vi "GOLPI full test.vi"() -> ()   [LabVIEW 2013, in "GOLPI library.lvlib"]
doc: "Makes test of all routines in GOLPI library. Good for testing changes in GOLPI library or testing compatibility with new versions of GNU Octave."
uses:
  GOLPI library.lvlib
  Set Variable - polymorph parts/Set Double.vi
  Get Variable - polymorph parts/Get Double.vi
  Set Variable - polymorph parts/Set Double Complex.vi
  Get Variable - polymorph parts/Get Double Complex.vi
  Set Variable - polymorph parts/Set 2D Array Double.vi
  Get Variable - polymorph parts/Get 2D Array Double.vi
  Set Variable - polymorph parts/Set 2D Array Double Complex.vi
  Get Variable - polymorph parts/Get 2D Array Double Complex.vi
  Set Variable - polymorph parts/Set String.vi
  Get Variable - polymorph parts/Get String.vi
  Set Variable - polymorph parts/Set 1D Array String.vi
  Get Variable - polymorph parts/Get 1D Array String.vi
panel:
  out "now running test no:":i32
  out "all tests result":bool
  out "test results":T1(array[cluster])
  in  "do tests with large random datasets?":bool
  out "GNU Octave version":string
  out "exit code":i32
  out "error out":errorcluster
  in  "Octave binary directory":path=path "C:/Program Files/Octave-3.6.2/bin"
  in  "Working directory":path=path "C:/"
  # "Runs various tests and checks all parts of GOLPI library.\nSelecting 'do tests with large random datasets' cause\nrunning of time consuming tests.\nIf all tests are OK, GOLPI is fully working with selected\nGNU Octave binary."
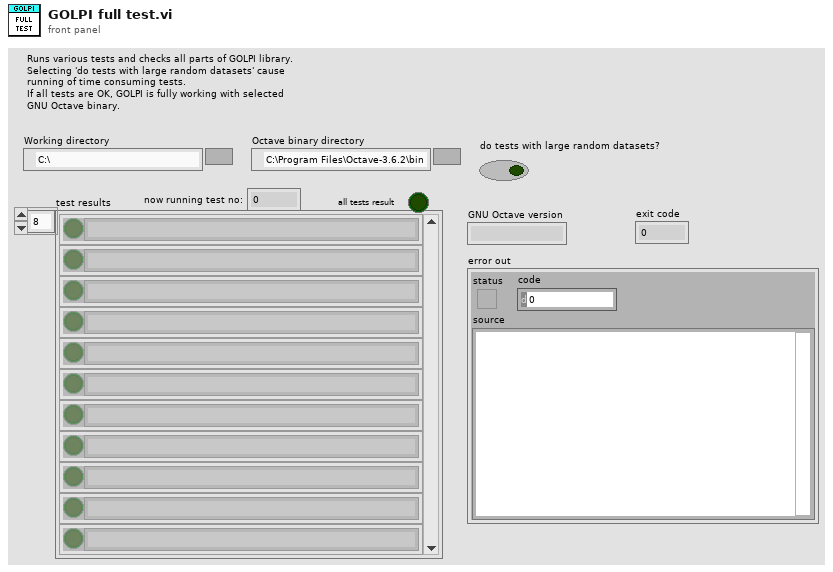
[diagram p1: front panel]
types:
  T1 = cluster{"test result":bool, "variable name":string}[]
  T2 = typedef "GOLPI library.lvlib/GOLPI reference Type Def.ctl" = cluster{"pipe handle":T3, "fast read timeout [ms]":u32, "fast read settle time [ms]":u32, "fast read to multiple [ms]":u32, "max elements per input line":u32, "slow read timeout [ms]":u32, "stdin double format specifier":string, "max elements per stdout output column":u32}
  T3 = typedef "LV Process library.lvlib/Pipe Handle.ctl" = cluster{"lv_proc.dll file path":path, "process instance handle":u32[]}
  T4 = cluster{"test result":bool, "variable name":string}
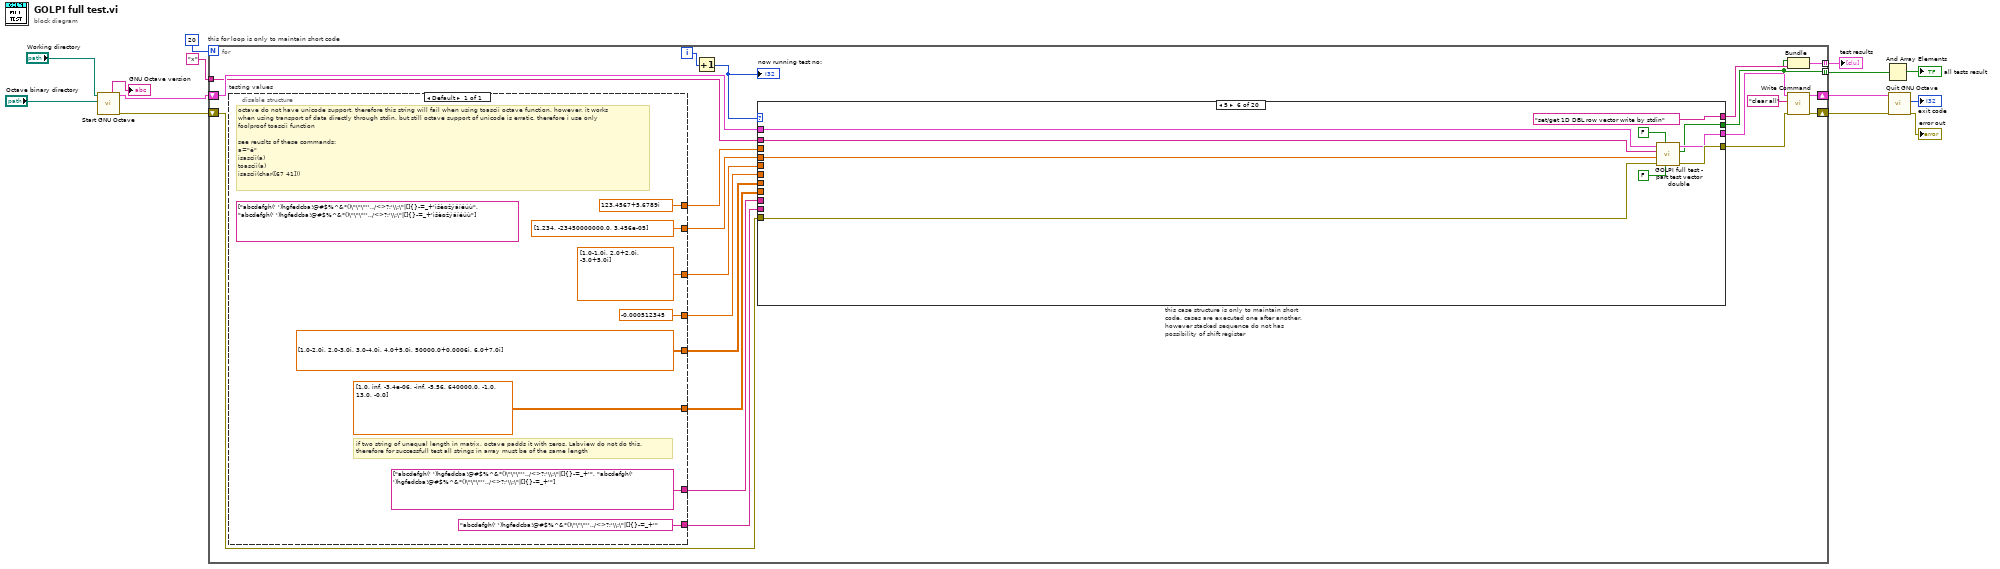
[diagram p0: block diagram]
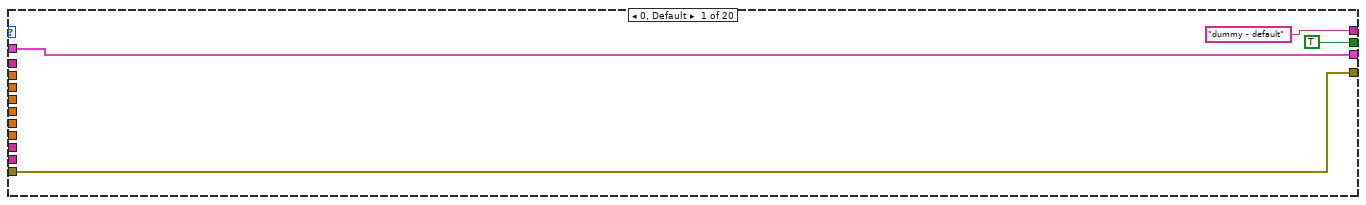
[diagram p2: hidden frame]
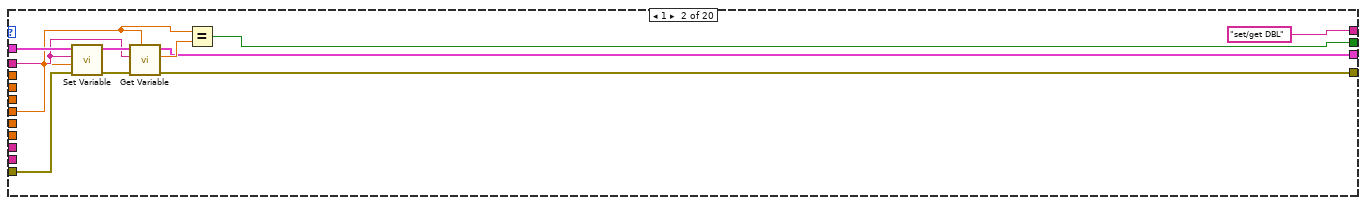
[diagram p3: hidden frame]
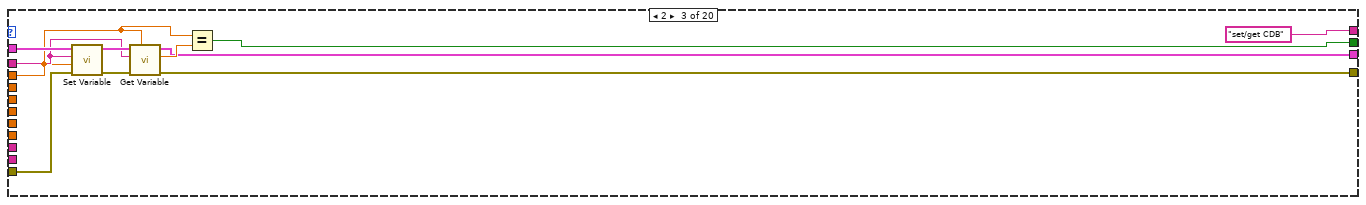
[diagram p4: hidden frame]
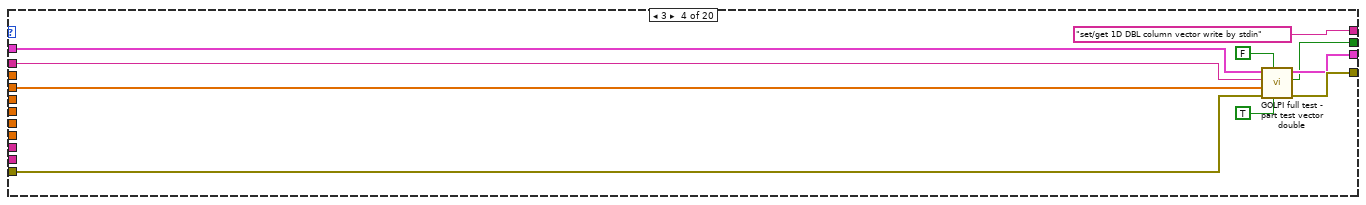
[diagram p5: hidden frame]
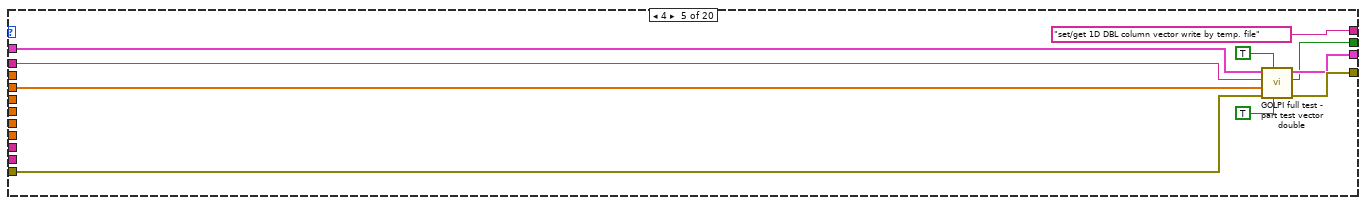
[diagram p6: hidden frame]
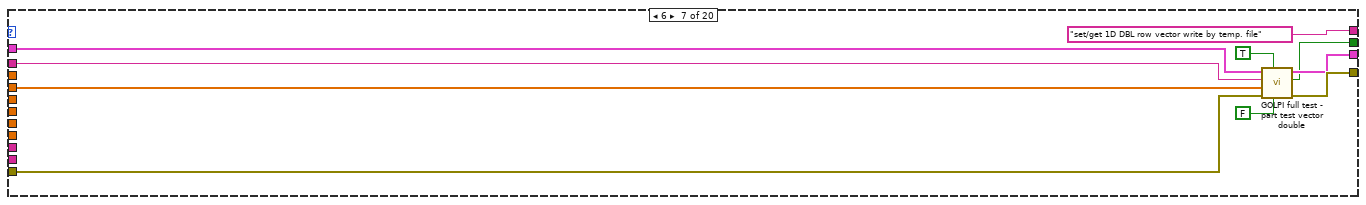
[diagram p7: hidden frame]
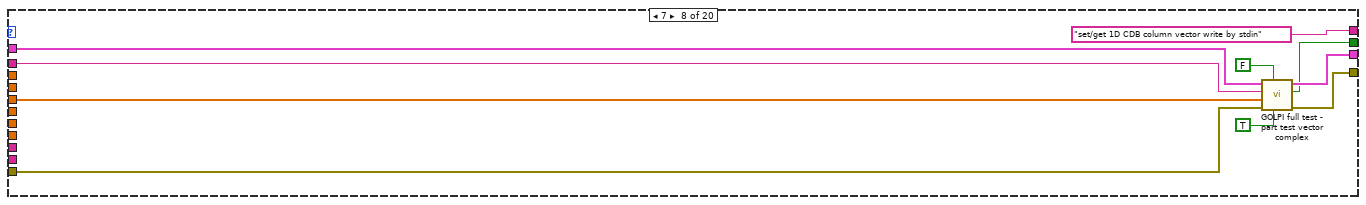
[diagram p8: hidden frame]
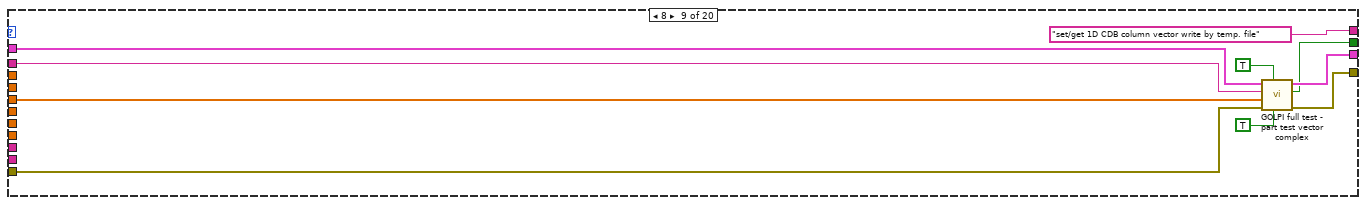
[diagram p9: hidden frame]
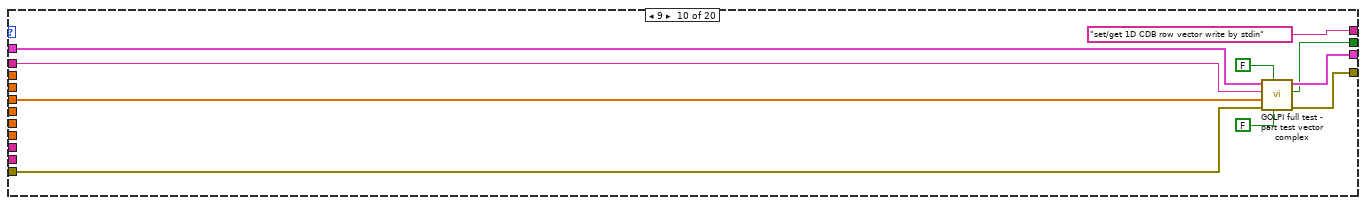
[diagram p10: hidden frame]
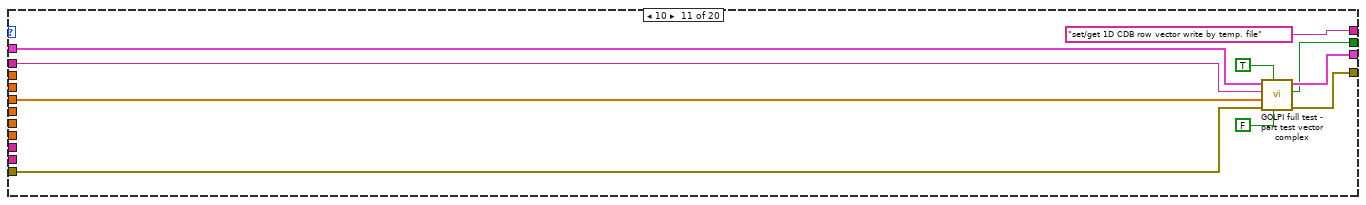
[diagram p11: hidden frame]
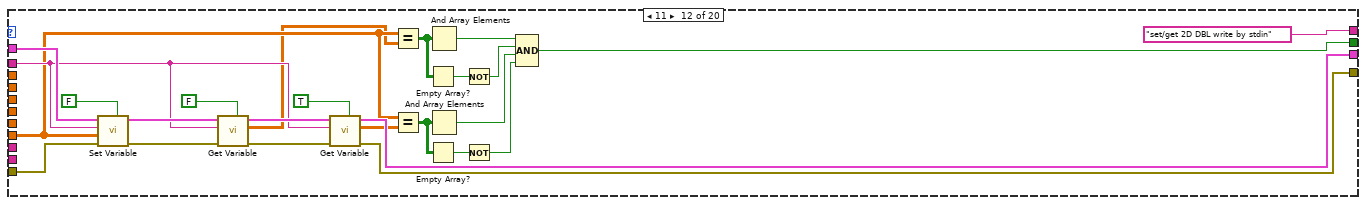
[diagram p12: hidden frame]
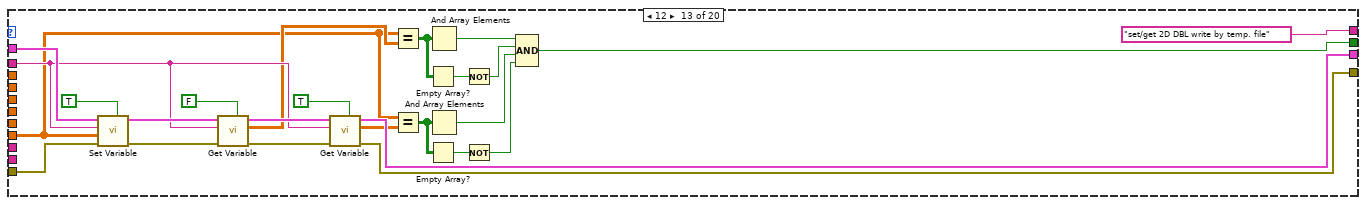
[diagram p13: hidden frame]
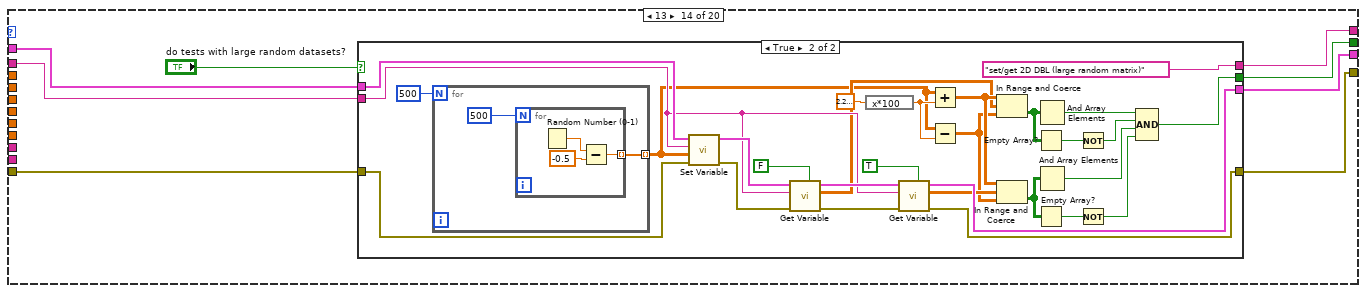
[diagram p14: hidden frame]
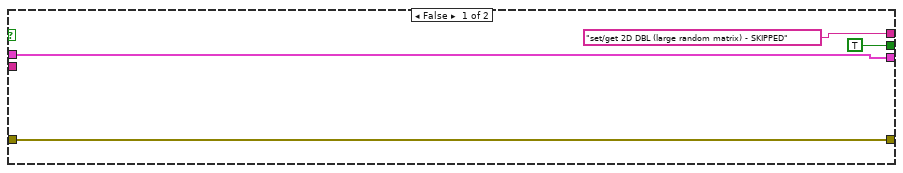
[diagram p15: hidden frame]
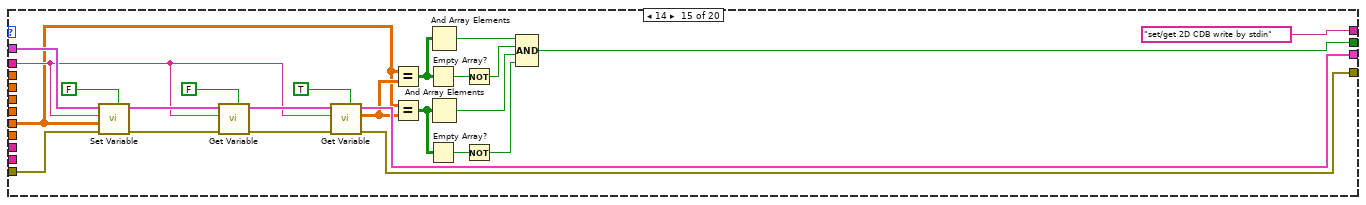
[diagram p16: hidden frame]
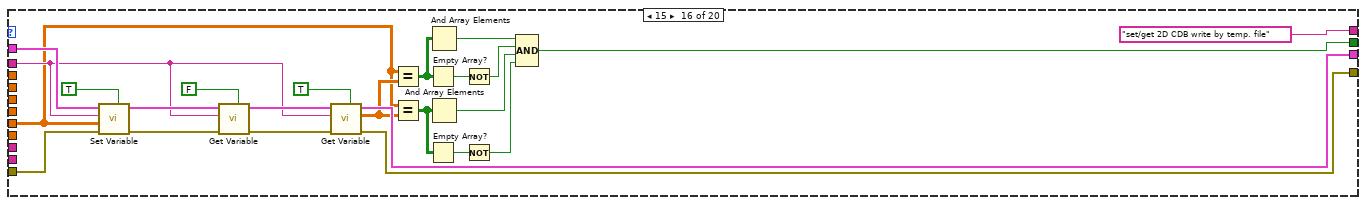
[diagram p17: hidden frame]
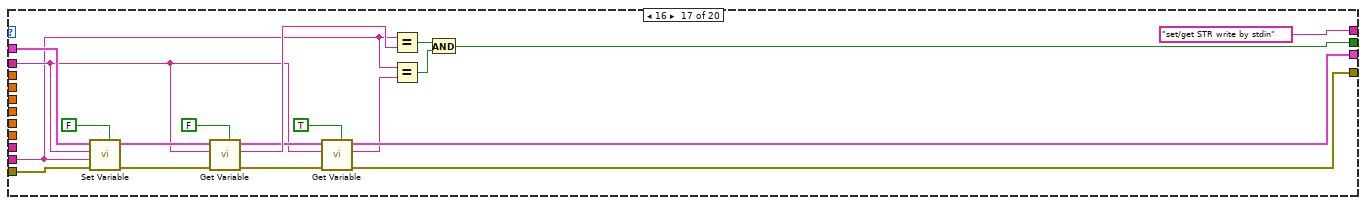
[diagram p18: hidden frame]
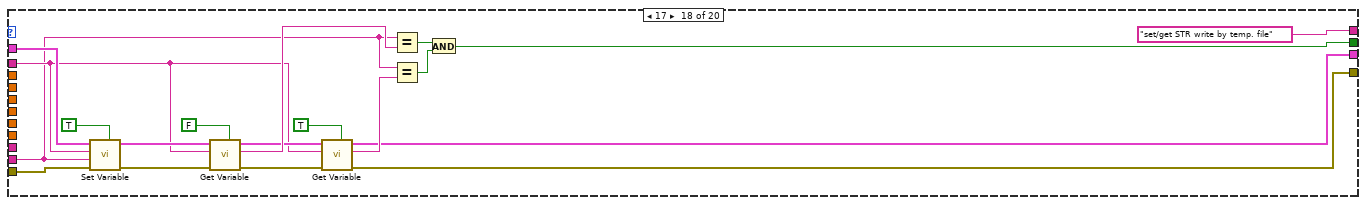
[diagram p19: hidden frame]
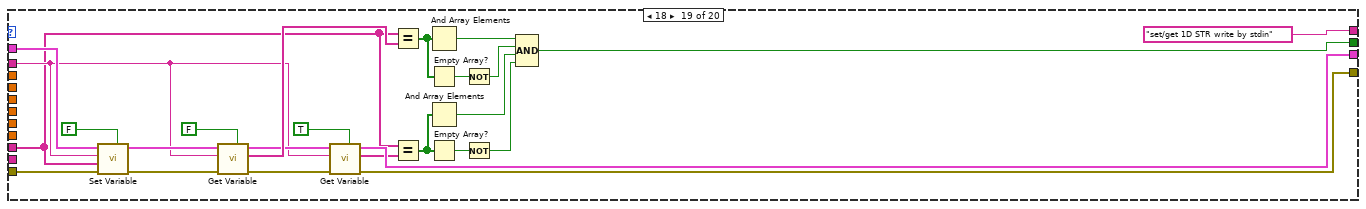
[diagram p20: hidden frame]
diagram:
  n1 = call "Start GNU Octave.vi"("Octave binary directory"="Octave binary directory", "Working directory"="Working directory") -> ("error out"=w9:errorcluster, "GOLPI ref. out"=w10:T2, "GNU Octave version"=→"GNU Octave version":string)  [unwired: 6 in, 1 out]
  n2 = for "this for loop is only to maintain short code" {
    N: 20 -> [_]
    tunnel: "x" ("variable name") -> [w33]
    shift-right: [w24] -> w6
    shift-left: w9 -> [w34]
    shift-right: [w26] -> w7
    shift-left: w10 -> [w35]
    tunnel: [w29] -> w4 mode=indexing
    tunnel: [w28] -> w3 mode=indexing
    i -> [w32]
    n3 = disable-structure "testing values" shown="Default" {
      disable-tunnel: [-0.000512345 ("value")] -> w22
      disable-tunnel: [dbl[] [1.234, -23450000000.0, 3.456e-05] ("value")] -> w21
      disable-tunnel: [cdb[] [1.0-1.0i, 2.0+2.0i, -3.0+5.0i] ("value")] -> w20
      disable-tunnel: [dbl[][] [[1.0, inf, -3.4e-06], [-inf, -5.56, 640000.0], [-1.0, 13.0, -0.0]] ("value")] -> w19
      disable-tunnel: [cdb[][] [[1.0-2.0i, 2.0-3.0i, 3.0-4.0i], [4.0+5.0i, 50000.0+0.0006i, 6.0+7.0i]] ("value")] -> w18
      disable-tunnel: ["abcdefgh(' ')hgfedcba!@#$%^&*()\"\"\"'',./<>?;'\\:\"|[]{}-=_+'" ("value")] -> w17
      disable-tunnel: [string[] ["abcdefgh(' ')hgfedcba!@#$%^&*()\"\"\"'',./<>?;'\\:\"|[]{}-=_+'", "abcdefgh(' ')hgfedcba!@#$%^&*()\"\"\"'',./<>?;'\\:\"|[]{}-=_+'"]] -> w16
      disable-tunnel: [cdb 123.4567+5.6789i ("value")] -> w15
      frame Enabled {
        (unwired) string[] ["abcdefgh(' ')hgfedcba!@#$%^&*()\"\"\"'',./<>?;'\\:\"|[]{}-=_+'ìšèøžýáíéúù", "abcdefgh(' ')hgfedcba!@#$%^&*()\"\"\"'',./<>?;'\\:\"|[]{}-=_+'ìšèøžýáíéúù"]
        # "octave do not have unicode support, therefore this string will fail when using toascii octave function. however, it works\nwhen using transport of data directly through stdin. but still octave support of unicode is erratic, therefore i use only\nfoolproof toascii function\n\nsee reuslts of these commands:\na=\"é\"\nisascii(a)\ntoascii(a)\nisascii(char([67 41]))"
        # "if two string of unequal length in matrix, octave padds it with zeros. Labview do not do this.\ntherefore for successfull test all strings in array must be of the same length"
      }
    }
    n4 = Increment(x=w32) -> (x+1=w31:i32)
    "now running test no:" <- w31
    n5 = case "this case structure is only to maintain short code. cases are executed one after another. however stacked sequence do not has possibility of shift register" shown="5" w31 {
      tunnel: w35 -> [w46 w55 w62 w75 w85 w97 w107 w119 w129 w136 w146 w170 w195 w203 w268 w292 w310 w329 w354 w379]
      tunnel: w34 -> [w47 w54 w63 w78 w88 w99 w109 w116 w126 w139 w149 w171 w196 w204 w269 w293 w311 w330 w355 w380]
      tunnel: [w47 w53 w64 w77 w87 w96 w106 w117 w127 w138 w148 w173 w198 w206 w267 w291 w303 w320 w342 w363] -> w25
      tunnel: [w46 w52 w65 w76 w86 w95 w105 w118 w128 w137 w147 w172 w197 w205 w266 w290 w304 w318 w341 w365] -> w27
      tunnel: w33 -> [_ w51 w61 w74 w84 w98 w108 w115 w125 w135 w145 w157 w182 w202 w248 w272 w301 w314 w340 w362]
      tunnel: [TRUE w50 w66 w71 w81 w94 w104 w113 w123 w132 w142 w174 w199 w207 w265 w289 w295 w316 w345 w370] -> w28
      tunnel: ["dummy - default" ("variable name") "set/get DBL" ("variable name") "set/get CDB" ("variable name") "set/get 1D DBL column vector write by stdin" ("variable name") "set/get 1D DBL column vector write by temp. file" ("variable name") "set/get 1D DBL row vector write by stdin" ("variable name") "set/get 1D DBL row vector write by temp. file" ("variable name") "set/get 1D CDB column vector write by stdin" ("variable name") "set/get 1D CDB column vector write by temp. file" ("variable name") "set/get 1D CDB row vector write by stdin" ("variable name") "set/get 1D CDB row vector write by temp. file" ("variable name") "set/get 2D DBL write by stdin" ("variable name") "set/get 2D DBL write by temp. file" ("variable name") w201 "set/get 2D CDB write by stdin" ("variable name") "set/get 2D CDB write by temp. file" ("variable name") "set/get STR write by stdin" ("variable name") "set/get STR write by temp. file" ("variable name") "set/get 1D STR write by stdin" ("variable name") "set/get 1D STR write by temp. file" ("variable name")] -> w30
      tunnel: w22 -> [_ w48 _ _ _ _ _ _ _ _ _ _ _ _ _ _ _ _ _ _]
      tunnel: w15 -> [_ _ w59 _ _ _ _ _ _ _ _ _ _ _ _ _ _ _ _ _]
      tunnel: w21 -> [_ _ _ w70 w80 w90 w100 _ _ _ _ _ _ _ _ _ _ _ _ _]
      tunnel: w20 -> [_ _ _ _ _ _ _ w110 w120 w130 w140 _ _ _ _ _ _ _ _ _]
      tunnel: w19 -> [_ _ _ _ _ _ _ _ _ _ _ w152 w175 _ _ _ _ _ _ _]
      tunnel: w18 -> [_ _ _ _ _ _ _ _ _ _ _ _ _ _ w246 w270 _ _ _ _]
      tunnel: w17 -> [_ _ _ _ _ _ _ _ _ _ _ _ _ _ _ _ w294 w313 _ _]
      tunnel: w16 -> [_ _ _ _ _ _ _ _ _ _ _ _ _ _ _ _ _ _ w332 w357]
      frame 0, Default {
      }
      frame 1 {
        n6 = call-poly "Set Variable.vi"("error in"=w54, "value"=w48, "variable name"=w51, "GOLPI ref. in"=w55) -> ("error out"=w57:errorcluster, "GOLPI ref. out"=w58:T2)  [unwired: 6 in]
        n7 = call-poly "Get Variable.vi"("data type of variable"=w48, "error in"=w57, "variable name"=w51, "GOLPI ref. in"=w58) -> ("error out"=w53:errorcluster, "value"=w56:dbl, "GOLPI ref. out"=w52:T2)  [unwired: 5 in]
        n8 = Equal?(x=w48, y=w56) -> (x = y?=w50:bool)
      }
      frame 2 {
        n9 = call-poly "Set Variable.vi"("error in"=w63, "value"=w59, "variable name"=w61, "GOLPI ref. in"=w62) -> ("error out"=w68:errorcluster, "GOLPI ref. out"=w67:T2)  [unwired: 6 in]
        n10 = call-poly "Get Variable.vi"("data type of variable"=w59, "error in"=w68, "variable name"=w61, "GOLPI ref. in"=w67) -> ("error out"=w64:errorcluster, "value"=w69:cdb, "GOLPI ref. out"=w65:T2)  [unwired: 5 in]
        n11 = Equal?(x=w59, y=w69) -> (x = y?=w66:bool)
      }
      frame 3 {
        n12 = call "GOLPI full test - part test vector double.vi"("column vector?"=TRUE, "set: use temporary file?"=FALSE, "error in (no error)"=w78, "test value"=w70, "variable name in"=w74, "GOLPI ref. in"=w75) -> ("error out"=w77:errorcluster, "test result"=w71:bool, "GOLPI ref. out"=w76:T2)  [unwired: 3 in]
      }
      frame 4 {
        n13 = call "GOLPI full test - part test vector double.vi"("column vector?"=TRUE, "set: use temporary file?"=TRUE, "error in (no error)"=w88, "test value"=w80, "variable name in"=w84, "GOLPI ref. in"=w85) -> ("error out"=w87:errorcluster, "test result"=w81:bool, "GOLPI ref. out"=w86:T2)  [unwired: 3 in]
      }
      frame 5 {
        n14 = call "GOLPI full test - part test vector double.vi"("column vector?"=FALSE, "set: use temporary file?"=FALSE, "error in (no error)"=w99, "test value"=w90, "variable name in"=w98, "GOLPI ref. in"=w97) -> ("error out"=w96:errorcluster, "test result"=w94:bool, "GOLPI ref. out"=w95:T2)  [unwired: 3 in]
      }
      frame 6 {
        n15 = call "GOLPI full test - part test vector double.vi"("column vector?"=FALSE, "set: use temporary file?"=TRUE, "error in (no error)"=w109, "test value"=w100, "variable name in"=w108, "GOLPI ref. in"=w107) -> ("error out"=w106:errorcluster, "test result"=w104:bool, "GOLPI ref. out"=w105:T2)  [unwired: 3 in]
      }
      frame 7 {
        n16 = call "GOLPI full test - part test vector complex.vi"("column vector?"=TRUE, "set: use temporary file?"=FALSE, "error in (no error)"=w116, "test value"=w110, "variable name in"=w115, "GOLPI ref. in"=w119) -> ("error out"=w117:errorcluster, "test result"=w113:bool, "GOLPI ref. out"=w118:T2)  [unwired: 3 in]
      }
      frame 8 {
        n17 = call "GOLPI full test - part test vector complex.vi"("column vector?"=TRUE, "set: use temporary file?"=TRUE, "error in (no error)"=w126, "test value"=w120, "variable name in"=w125, "GOLPI ref. in"=w129) -> ("error out"=w127:errorcluster, "test result"=w123:bool, "GOLPI ref. out"=w128:T2)  [unwired: 3 in]
      }
      frame 9 {
        n18 = call "GOLPI full test - part test vector complex.vi"("column vector?"=FALSE, "set: use temporary file?"=FALSE, "error in (no error)"=w139, "test value"=w130, "variable name in"=w135, "GOLPI ref. in"=w136) -> ("error out"=w138:errorcluster, "test result"=w132:bool, "GOLPI ref. out"=w137:T2)  [unwired: 3 in]
      }
      frame 10 {
        n19 = call "GOLPI full test - part test vector complex.vi"("column vector?"=FALSE, "set: use temporary file?"=TRUE, "error in (no error)"=w149, "test value"=w140, "variable name in"=w145, "GOLPI ref. in"=w146) -> ("error out"=w148:errorcluster, "test result"=w142:bool, "GOLPI ref. out"=w147:T2)  [unwired: 3 in]
      }
      frame 11 {
        n20 = call-poly "Set Variable.vi"("use temporary file? (F)"=FALSE ("use temporary file?"), "error in"=w171, "value"=w152, "variable name"=w157, "GOLPI ref. in"=w170) -> ("error out"=w161:errorcluster, "GOLPI ref. out"=w159:T2)  [unwired: 5 in]
        n21 = call-poly "Get Variable.vi"("use temporary file? (F)"=FALSE ("use temporary file?"), "error in"=w161, "variable name"=w157, "GOLPI ref. in"=w159) -> ("error out"=w160:errorcluster, "value"=w151:dbl[][], "GOLPI ref. out"=w158:T2)  [unwired: 5 in]
        n22 = call-poly "Get Variable.vi"("use temporary file? (F)"=TRUE ("use temporary file?"), "error in"=w160, "variable name"=w157, "GOLPI ref. in"=w158) -> ("error out"=w173:errorcluster, "value"=w163:dbl[][], "GOLPI ref. out"=w172:T2)  [unwired: 5 in]
        n23 = Equal?(x=w152, y=w151) -> (x = y?=w150:bool[][])
        n24 = Equal?(x=w152, y=w163) -> (x = y?=w165:bool[][])
        n25 = Empty Array?(array=w150) -> (empty?=w155:bool)
        n26 = Empty Array?(array=w165) -> (empty?=w166:bool)
        n27 = And Array Elements(Boolean array=w150) -> (logical AND=w156:bool)
        n28 = And Array Elements(Boolean array=w165) -> (logical AND=w168:bool)
        n29 = Not(x=w155) -> (.not. x?=w154:bool)
        n30 = Not(x=w166) -> (.not. x?=w167:bool)
        n31 = Compound Arithmetic op=AND(w156, w154, w168, w167) -> (w174:bool)
      }
      frame 12 {
        n32 = call-poly "Set Variable.vi"("use temporary file? (F)"=TRUE ("use temporary file?"), "error in"=w196, "value"=w175, "variable name"=w182, "GOLPI ref. in"=w195) -> ("error out"=w186:errorcluster, "GOLPI ref. out"=w184:T2)  [unwired: 5 in]
        n33 = call-poly "Get Variable.vi"("use temporary file? (F)"=FALSE ("use temporary file?"), "error in"=w186, "variable name"=w182, "GOLPI ref. in"=w184) -> ("error out"=w185:errorcluster, "value"=w180:dbl[][], "GOLPI ref. out"=w183:T2)  [unwired: 5 in]
        n34 = call-poly "Get Variable.vi"("use temporary file? (F)"=TRUE ("use temporary file?"), "error in"=w185, "variable name"=w182, "GOLPI ref. in"=w183) -> ("error out"=w198:errorcluster, "value"=w188:dbl[][], "GOLPI ref. out"=w197:T2)  [unwired: 5 in]
        n35 = Equal?(x=w175, y=w180) -> (x = y?=w181:bool[][])
        n36 = Equal?(x=w175, y=w188) -> (x = y?=w190:bool[][])
        n37 = Empty Array?(array=w181) -> (empty?=w178:bool)
        n38 = Empty Array?(array=w190) -> (empty?=w191:bool)
        n39 = And Array Elements(Boolean array=w181) -> (logical AND=w179:bool)
        n40 = And Array Elements(Boolean array=w190) -> (logical AND=w193:bool)
        n41 = Not(x=w178) -> (.not. x?=w177:bool)
        n42 = Not(x=w191) -> (.not. x?=w192:bool)
        n43 = Compound Arithmetic op=AND(w179, w177, w193, w192) -> (w199:bool)
      }
      frame 13 {
        n44 = case shown="True" "do tests with large random datasets?" {
          tunnel: [TRUE w236] -> w207
          tunnel: [w211 w235] -> w206
          tunnel: [w210 w234] -> w205
          tunnel: w204 -> [w211 w233]
          tunnel: w203 -> [w210 w232]
          tunnel: w202 -> [_ w218]
          tunnel: ["set/get 2D DBL (large random matrix) - SKIPPED" ("variable name") "set/get 2D DBL (large random matrix)" ("variable name")] -> w201
          frame False {
          }
          frame True {
            n45 = for {
              N: 500 ("dimension size") -> [_]
              tunnel: [w242] -> w212 mode=indexing
              n46 = for {
                N: 500 ("dimension size") -> [_]
                tunnel: [w243] -> w242 mode=indexing
                n47 = Random Number (0-1)() -> (number: 0 to 1=w245:dbl)
                n48 = Subtract(x=w245, y=-0.5) -> (x-y=w243:dbl)
              }
            }
            n49 = call-poly "Set Variable.vi"("error in"=w233, "value"=w212, "variable name"=w218, "GOLPI ref. in"=w232) -> ("error out"=w224:errorcluster, "GOLPI ref. out"=w227:T2)  [unwired: 6 in]
            n50 = call-poly "Get Variable.vi"("use temporary file? (F)"=FALSE ("use temporary file?"), "error in"=w224, "variable name"=w218, "GOLPI ref. in"=w227) -> ("error out"=w225:errorcluster, "value"=w217:dbl[][], "GOLPI ref. out"=w226:T2)  [unwired: 5 in]
            n51 = expression code="x*100"(2.220446049250313e-16) -> (w215:dbl)
            n52 = call-poly "Get Variable.vi"("use temporary file? (F)"=TRUE ("use temporary file?"), "error in"=w225, "variable name"=w218, "GOLPI ref. in"=w226) -> ("error out"=w235:errorcluster, "value"=w229:dbl[][], "GOLPI ref. out"=w234:T2)  [unwired: 5 in]
            n53 = Add(x=w212, y=w215) -> (x+y=w222:dbl[][])
            n54 = Subtract(x=w212, y=w215) -> (x-y=w213:dbl[][])
            n55 = In Range and Coerce(upper limit=w222, x=w217, lower limit=w213) -> (In Range?=w214:bool[][])  [unwired: 1 out]
            n56 = In Range and Coerce(upper limit=w222, x=w229, lower limit=w213) -> (In Range?=w228:bool[][])  [unwired: 1 out]
            n57 = Empty Array?(array=w214) -> (empty?=w221:bool)
            n58 = Empty Array?(array=w228) -> (empty?=w238:bool)
            n59 = And Array Elements(Boolean array=w214) -> (logical AND=w220:bool)
            n60 = And Array Elements(Boolean array=w228) -> (logical AND=w240:bool)
            n61 = Not(x=w221) -> (.not. x?=w219:bool)
            n62 = Not(x=w238) -> (.not. x?=w239:bool)
            n63 = Compound Arithmetic op=AND(w220, w219, w240, w239) -> (w236:bool)
          }
        }
      }
      frame 14 {
        n64 = call-poly "Set Variable.vi"("use temporary file? (F)"=FALSE ("use temporary file?"), "error in"=w269, "value"=w246, "variable name"=w248, "GOLPI ref. in"=w268) -> ("error out"=w256:errorcluster, "GOLPI ref. out"=w257:T2)  [unwired: 5 in]
        n65 = call-poly "Get Variable.vi"("use temporary file? (F)"=FALSE ("use temporary file?"), "error in"=w256, "variable name"=w248, "GOLPI ref. in"=w257) -> ("error out"=w254:errorcluster, "GOLPI ref. out"=w255:T2)  [unwired: 5 in, 1 out]
        n66 = call-poly "Get Variable.vi"("use temporary file? (F)"=TRUE ("use temporary file?"), "error in"=w254, "variable name"=w248, "GOLPI ref. in"=w255) -> ("error out"=w267:errorcluster, "value"=w249:cdb[][], "GOLPI ref. out"=w266:T2)  [unwired: 5 in]
        n67 = Equal?(x=w246, y=w249) -> (x = y?=w252:bool[][])
        n68 = Equal?(x=w246, y=w249) -> (x = y?=w262:bool[][])
        n69 = Empty Array?(array=w252) -> (empty?=w253:bool)
        n70 = Empty Array?(array=w262) -> (empty?=w261:bool)
        n71 = And Array Elements(Boolean array=w252) -> (logical AND=w251:bool)
        n72 = And Array Elements(Boolean array=w262) -> (logical AND=w259:bool)
        n73 = Not(x=w253) -> (.not. x?=w250:bool)
        n74 = Not(x=w261) -> (.not. x?=w260:bool)
        n75 = Compound Arithmetic op=AND(w251, w250, w259, w260) -> (w265:bool)
      }
      frame 15 {
        n76 = call-poly "Set Variable.vi"("use temporary file? (F)"=TRUE ("use temporary file?"), "error in"=w293, "value"=w270, "variable name"=w272, "GOLPI ref. in"=w292) -> ("error out"=w280:errorcluster, "GOLPI ref. out"=w281:T2)  [unwired: 5 in]
        n77 = call-poly "Get Variable.vi"("use temporary file? (F)"=FALSE ("use temporary file?"), "error in"=w280, "variable name"=w272, "GOLPI ref. in"=w281) -> ("error out"=w278:errorcluster, "GOLPI ref. out"=w279:T2)  [unwired: 5 in, 1 out]
        n78 = call-poly "Get Variable.vi"("use temporary file? (F)"=TRUE ("use temporary file?"), "error in"=w278, "variable name"=w272, "GOLPI ref. in"=w279) -> ("error out"=w291:errorcluster, "value"=w273:cdb[][], "GOLPI ref. out"=w290:T2)  [unwired: 5 in]
        n79 = Equal?(x=w270, y=w273) -> (x = y?=w276:bool[][])
        n80 = Equal?(x=w270, y=w273) -> (x = y?=w286:bool[][])
        n81 = Empty Array?(array=w276) -> (empty?=w277:bool)
        n82 = Empty Array?(array=w286) -> (empty?=w285:bool)
        n83 = And Array Elements(Boolean array=w276) -> (logical AND=w275:bool)
        n84 = And Array Elements(Boolean array=w286) -> (logical AND=w283:bool)
        n85 = Not(x=w277) -> (.not. x?=w274:bool)
        n86 = Not(x=w285) -> (.not. x?=w284:bool)
        n87 = Compound Arithmetic op=AND(w275, w274, w283, w284) -> (w289:bool)
      }
      frame 16 {
        n88 = call-poly "Set Variable.vi"("use temporary file? (F)"=FALSE ("use temporary file?"), "error in"=w311, "value"=w294, "variable name"=w301, "GOLPI ref. in"=w310) -> ("error out"=w312:errorcluster, "GOLPI ref. out"=w309:T2)  [unwired: 5 in]
        n89 = call-poly "Get Variable.vi"("use temporary file? (F)"=FALSE ("use temporary file?"), "error in"=w312, "variable name"=w301, "GOLPI ref. in"=w309) -> ("error out"=w302:errorcluster, "value"=w308:string, "GOLPI ref. out"=w305:T2)  [unwired: 5 in]
        n90 = call-poly "Get Variable.vi"("use temporary file? (F)"=TRUE ("use temporary file?"), "error in"=w302, "variable name"=w301, "GOLPI ref. in"=w305) -> ("error out"=w303:errorcluster, "value"=w298:string, "GOLPI ref. out"=w304:T2)  [unwired: 5 in]
        n91 = Equal?(x=w294, y=w308) -> (x = y?=w296:bool)
        n92 = Equal?(x=w294, y=w298) -> (x = y?=w297:bool)
        n93 = And(x=w296, y=w297) -> (x .and. y?=w295:bool)
      }
      frame 17 {
        n94 = call-poly "Set Variable.vi"("use temporary file? (F)"=TRUE ("use temporary file?"), "error in"=w330, "value"=w313, "variable name"=w314, "GOLPI ref. in"=w329) -> ("error out"=w331:errorcluster, "GOLPI ref. out"=w328:T2)  [unwired: 5 in]
        n95 = call-poly "Get Variable.vi"("use temporary file? (F)"=FALSE ("use temporary file?"), "error in"=w331, "variable name"=w314, "GOLPI ref. in"=w328) -> ("error out"=w321:errorcluster, "value"=w327:string, "GOLPI ref. out"=w319:T2)  [unwired: 5 in]
        n96 = call-poly "Get Variable.vi"("use temporary file? (F)"=TRUE ("use temporary file?"), "error in"=w321, "variable name"=w314, "GOLPI ref. in"=w319) -> ("error out"=w320:errorcluster, "value"=w323:string, "GOLPI ref. out"=w318:T2)  [unwired: 5 in]
        n97 = Equal?(x=w313, y=w327) -> (x = y?=w317:bool)
        n98 = Equal?(x=w313, y=w323) -> (x = y?=w322:bool)
        n99 = And(x=w317, y=w322) -> (x .and. y?=w316:bool)
      }
      frame 18 {
        n100 = call-poly "Set Variable.vi"("use temporary file? (F)"=FALSE ("use temporary file? 2"), "error in"=w355, "value"=w332, "variable name"=w340, "GOLPI ref. in"=w354) -> ("error out"=w356:errorcluster, "GOLPI ref. out"=w353:T2)  [unwired: 5 in]
        n101 = call-poly "Get Variable.vi"("use temporary file? (F)"=FALSE ("use temporary file?"), "error in"=w356, "variable name"=w340, "GOLPI ref. in"=w353) -> ("error out"=w343:errorcluster, "value"=w352:string[], "GOLPI ref. out"=w344:T2)  [unwired: 5 in]
        n102 = call-poly "Get Variable.vi"("use temporary file? (F)"=TRUE ("use temporary file?"), "error in"=w343, "variable name"=w340, "GOLPI ref. in"=w344) -> ("error out"=w342:errorcluster, "value"=w335:string[], "GOLPI ref. out"=w341:T2)  [unwired: 5 in]
        n103 = Equal?(x=w332, y=w352) -> (x = y?=w346:bool[])
        n104 = Equal?(x=w332, y=w335) -> (x = y?=w339:bool[])
        n105 = And Array Elements(Boolean array=w346) -> (logical AND=w349:bool)
        n106 = Empty Array?(array=w346) -> (empty?=w347:bool)
        n107 = And Array Elements(Boolean array=w339) -> (logical AND=w336:bool)
        n108 = Empty Array?(array=w339) -> (empty?=w338:bool)
        n109 = Not(x=w347) -> (.not. x?=w348:bool)
        n110 = Not(x=w338) -> (.not. x?=w337:bool)
        n111 = Compound Arithmetic op=AND(w349, w348, w336, w337) -> (w345:bool)
      }
      frame 19 {
        n112 = call-poly "Set Variable.vi"("use temporary file? (F)"=TRUE ("use temporary file? 2"), "error in"=w380, "value"=w357, "variable name"=w362, "GOLPI ref. in"=w379) -> ("error out"=w381:errorcluster, "GOLPI ref. out"=w378:T2)  [unwired: 5 in]
        n113 = call-poly "Get Variable.vi"("use temporary file? (F)"=FALSE ("use temporary file?"), "error in"=w381, "variable name"=w362, "GOLPI ref. in"=w378) -> ("error out"=w364:errorcluster, "value"=w377:string[], "GOLPI ref. out"=w366:T2)  [unwired: 5 in]
        n114 = call-poly "Get Variable.vi"("use temporary file? (F)"=TRUE ("use temporary file?"), "error in"=w364, "variable name"=w362, "GOLPI ref. in"=w366) -> ("error out"=w363:errorcluster, "value"=w358:string[], "GOLPI ref. out"=w365:T2)  [unwired: 5 in]
        n115 = Equal?(x=w357, y=w377) -> (x = y?=w371:bool[])
        n116 = Equal?(x=w357, y=w358) -> (x = y?=w367:bool[])
        n117 = And Array Elements(Boolean array=w371) -> (logical AND=w374:bool)
        n118 = Empty Array?(array=w371) -> (empty?=w372:bool)
        n119 = And Array Elements(Boolean array=w367) -> (logical AND=w361:bool)
        n120 = Empty Array?(array=w367) -> (empty?=w368:bool)
        n121 = Not(x=w372) -> (.not. x?=w373:bool)
        n122 = Not(x=w368) -> (.not. x?=w360:bool)
        n123 = Compound Arithmetic op=AND(w374, w373, w361, w360) -> (w370:bool)
      }
    }
    n124 = Bundle("test result"=w28, "variable name"=w30) -> (w29:T4)  [unwired: 1 in]
    n125 = call "Write Command.vi"("error in"=w25, "command"="clear all", "GOLPI ref. in"=w27) -> ("error out"=w24:errorcluster, "GOLPI ref. out"=w26:T2)  [unwired: 7 in]
  }
  "test results" <- w4
  n126 = And Array Elements(Boolean array=w3) -> (logical AND=→"all tests result":bool)
  n127 = call "Quit GNU Octave.vi"("error in"=w6, "GOLPI ref. in"=w7) -> ("error out"=→"error out":errorcluster, "exit code"=→"exit code":i32)  [unwired: 8 in]
